vi "Generate Square Wave.vi"(0 "Laser Control":T1 {"f0" format="%.32g"}) -> (14 "SW Out":i16)   [LabVIEW 2018]
uses:
  <vilib>/rvi/FXPMathLib/FxpMul/XNode/nifxpmath_Multiplier.xnode
  <vilib>/rvi/FXPMathLib/sim/FxpSim.dll
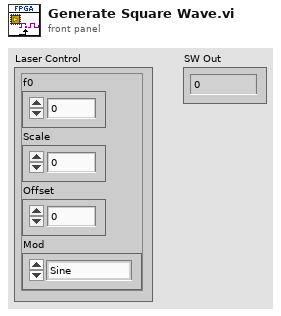
[diagram p1: front panel]
types:
  T1 = cluster{"f0":fxp<+,32,0>, "Scale":fxp<+,32,0>, "Offset":i16, "Mod":enum8{"Sine", "Square"}}
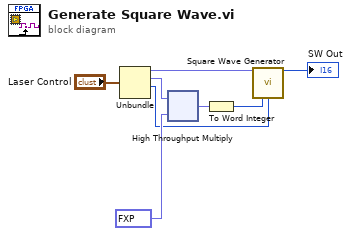
[diagram p0: block diagram]
diagram:
  n1 = Unbundle("Laser Control") -> ("f0"=w5:fxp<+,32,0>, "Scale"=w6:fxp<+,32,0>, "Offset"=w7:i16)  [unwired: 1 out]
  n2 = xnode ("High Throughput Multiply")("x"=w6, "y"=fxp<+,15,15> 32767.0 ("n")) -> ("x*y"=w2:fxp<+,47,15>)
  n3 = To Word Integer(number=w2) -> (16bit integer=w1:i16)
  n4 = call "Square Wave Generator"("frequency (periods/tick)"=w5, "amplitude"=w1, "offset"=w7) -> ("square wave out"=→"SW Out":i16)  [unwired: 12 in]
